vi "LEDExecute.vi"() -> ()   [LabVIEW 2023]
uses:
  <vilib>/Rock Robotics/WPI/DriverStation/WPI_DriverStationAllianceInfo.ctl
  Human/HumanGlobal.vi
  <vilib>/Rock Robotics/WPI/ThirdParty/PhotonVisionLib/PhotonVisionLib.lvlib
panel:
  out "Numeric":i32
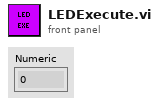
[diagram p1: front panel]
types:
  T1 = typedef "WPI_DriverStationAllianceInfo.ctl" = enum16{"Red", "Blue", "Invalid"}
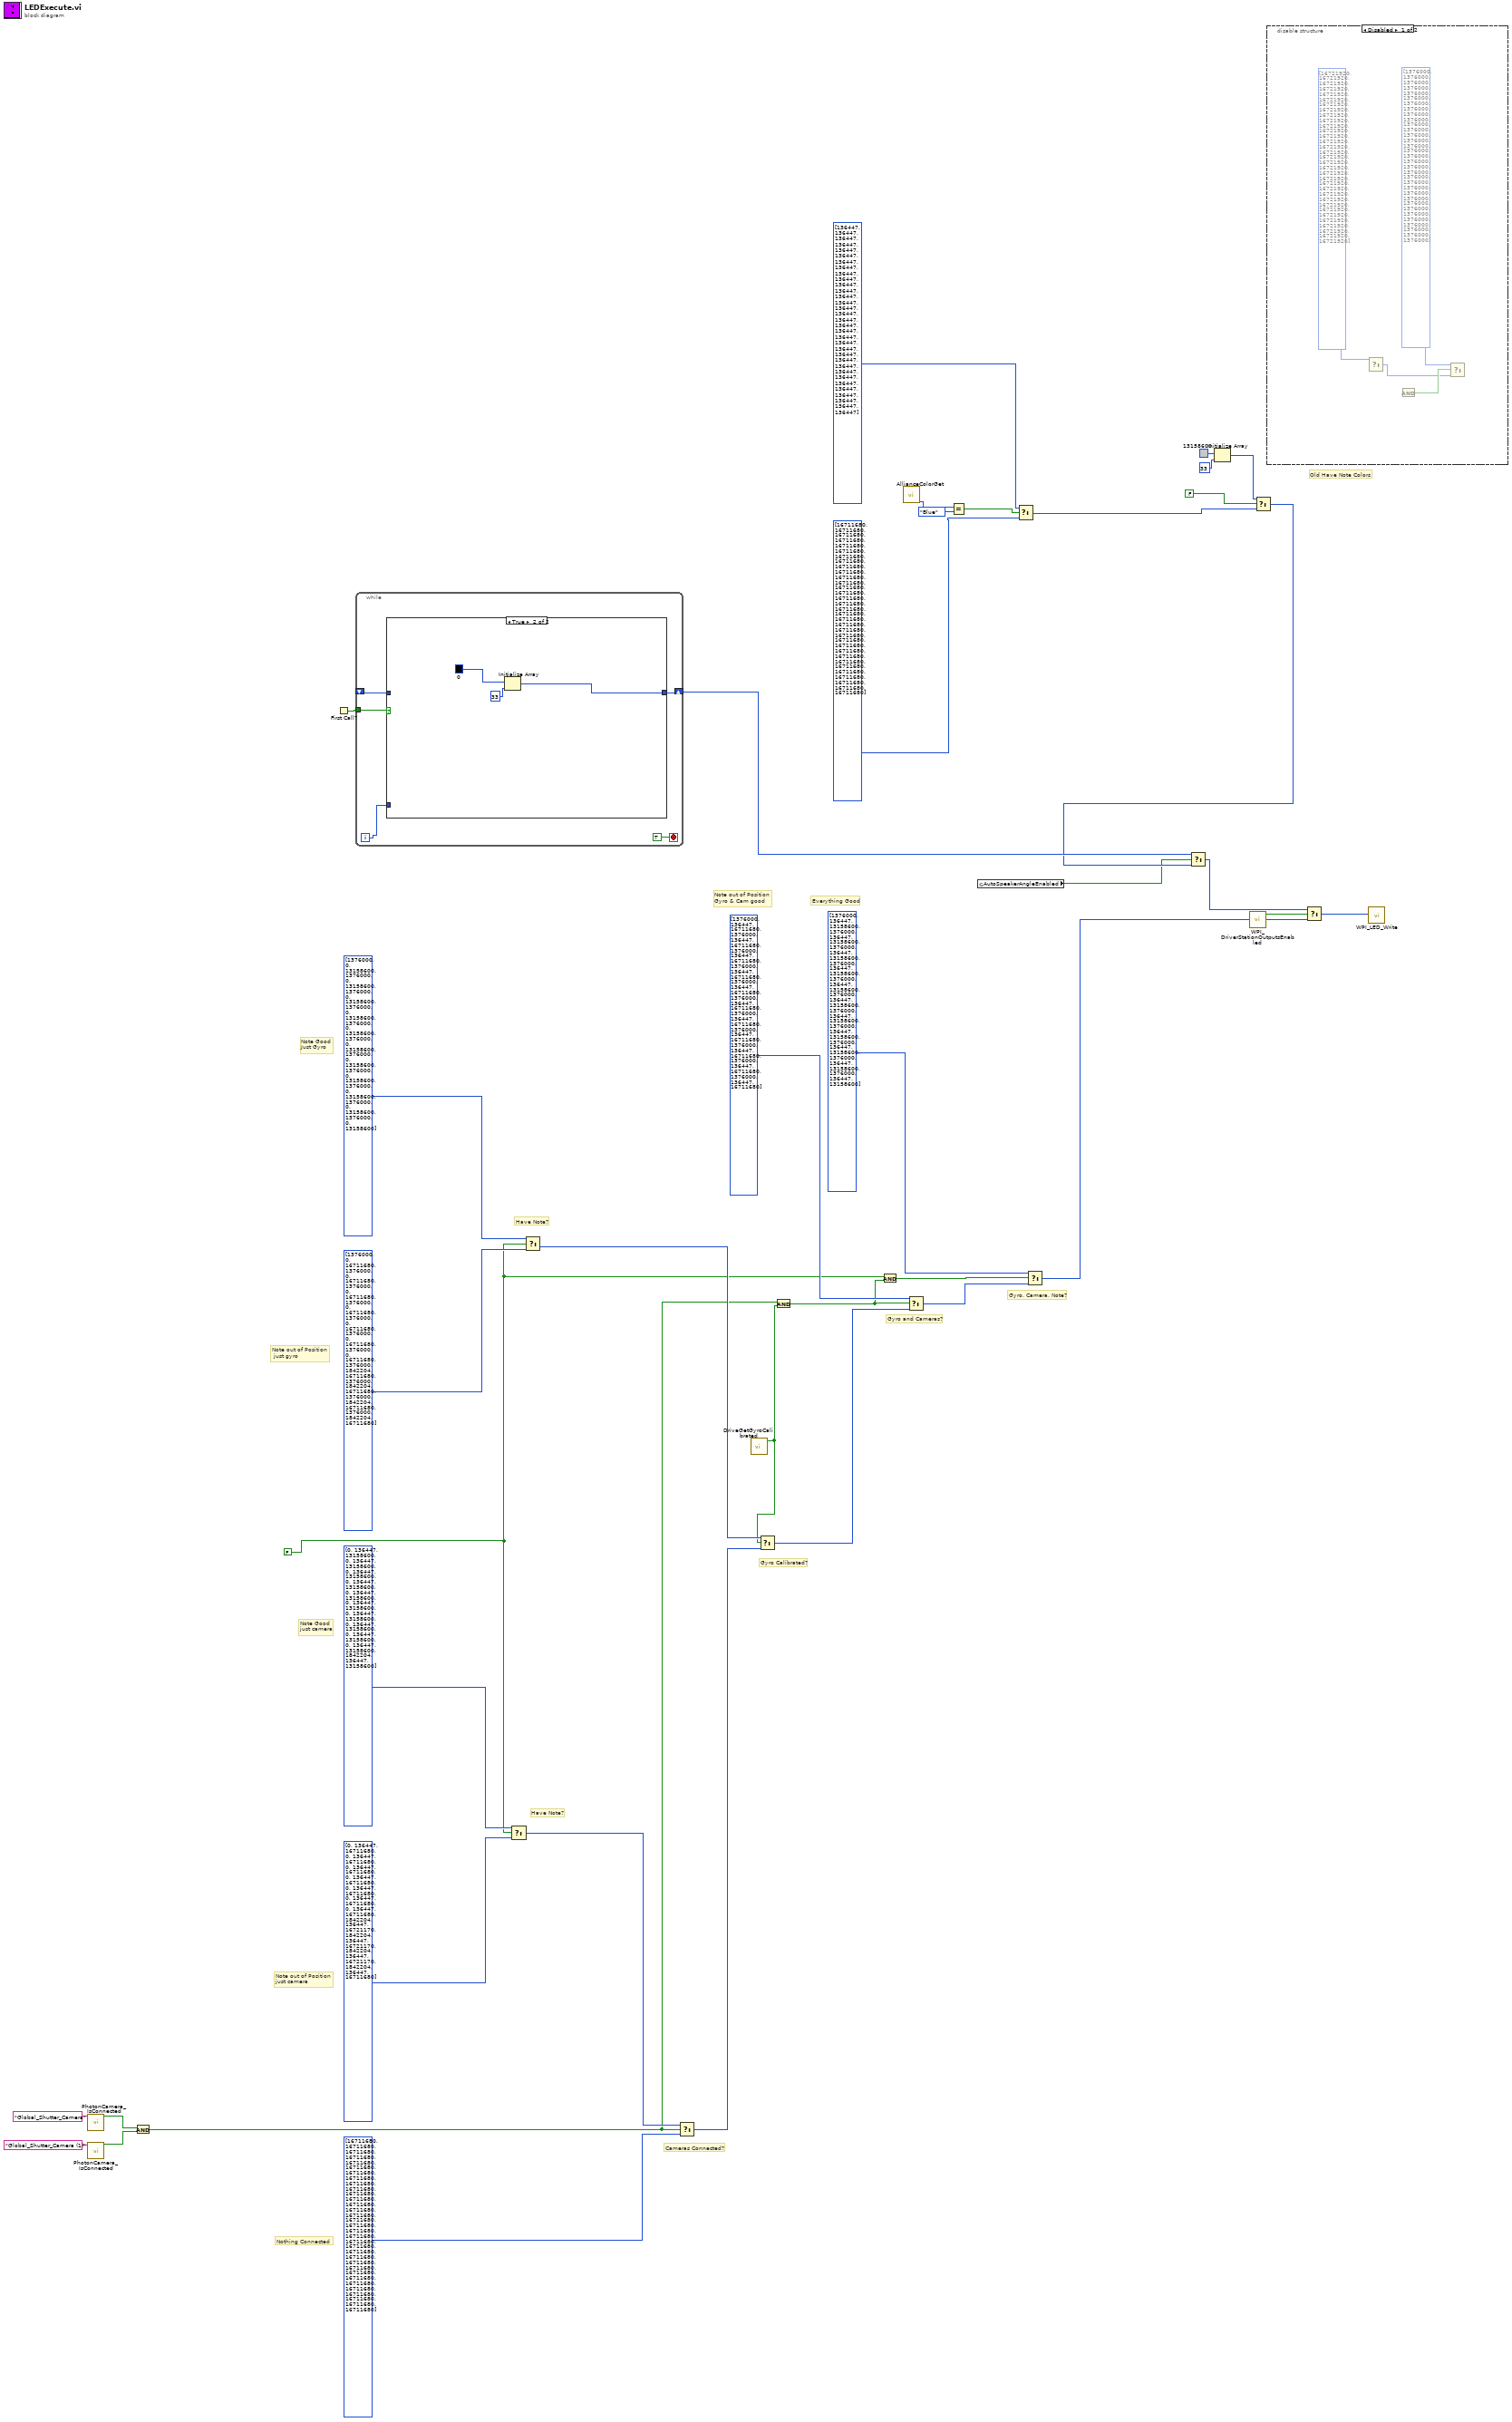
[diagram p0: block diagram]
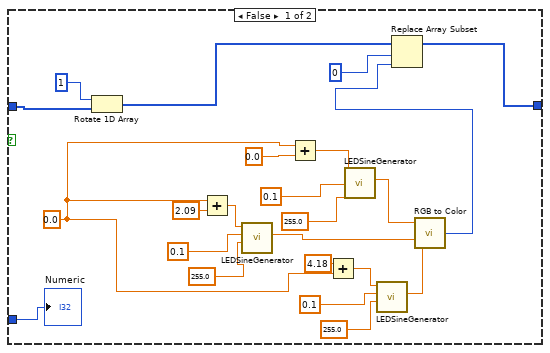
[diagram p2: hidden frame]
diagram:
  w1 = FALSE ("s")
  # "Old Have Note Colors"
  # "Gyro, Camera, Note?"
  # "Gyro and Cameras?"
  # "Gyro Calibrated?"
  # "Cameras Connected?"
  # "Have Note?"
  # "Have Note?"
  # "Note Good\njust camera"
  # "Note Good\nJust Gyro"
  # "Note out of Position\n just gyro"
  # "Note out of Position\njust camera"
  # "Everything Good"
  # "Note out of Position\nGyro & Cam good"
  # "Nothing Connected"
  n1 = call <vilib>:"PhotonCamera_IsConnected.vi"("CameraName"="Global_Shutter_Camera") -> ("IsConnected"=w20:bool)  [unwired: 9 in, 1 out]
  n2 = call <vilib>:"PhotonCamera_IsConnected.vi"("CameraName"="Global_Shutter_Camera (1)") -> ("IsConnected"=w19:bool)  [unwired: 9 in, 1 out]
  n3 = And(x=w20, y=w19) -> (x .and. y?=w23:bool)
  n4 = First Call?() -> (First Call?: T/F=w11:bool)
  n5 = while {
    tunnel: w11 -> [w43]
    shift-right: [w42] -> w9
    shift-left: _ -> [w41]
    i -> [w40]
    stop <- TRUE stop-if-true
    n6 = case shown="True" w43 {
      tunnel: [w58 w68] -> w42
      tunnel: w41 -> [w67 _]
      tunnel: w40 -> [w57 _]
      frame False {
        w61 = 0.0
        n7 = Rotate 1D Array(1:w67, 2:1 ("n")) -> (0:w65:u32[])
        n8 = Add(x=w61, y=2.09 ("Speed")) -> (x+y=w52:dbl)
        n9 = call "LEDSineGenerator.vi"("Amplitude"=255.0, "Speed"=0.1 ("Delay"), "Delay"=w52) -> ("Output"=w49:dbl)  [unwired: 8 in]
        n10 = Add(x=w61, y=0.0 ("Speed")) -> (x+y=w56:dbl)
        n11 = Add(x=4.18 ("Speed"), y=w61) -> (x+y=w48:dbl)
        n12 = call "LEDSineGenerator.vi"("Amplitude"=255.0, "Speed"=0.1 ("Delay"), "Delay"=w56) -> ("Output"=w53:dbl)  [unwired: 8 in]
        n13 = call "LEDSineGenerator.vi"("Amplitude"=255.0, "Speed"=0.1 ("Delay"), "Delay"=w48) -> ("Output"=w45:dbl)  [unwired: 8 in]
        n14 = call <vilib>:"RGB to Color.vi"("B"=w45, "G"=w49, "R"=w53) -> ("Color"=w60:u32)
        n15 = Replace Array Subset(array=w65, new element=w60, index=0) -> (w58:u32[])
        "Numeric" <- w57
      }
      frame True {
        n16 = Initialize Array(u32 0 ("Color Box 3"), 33 ("dimension size")) -> (w68:u32[])
      }
    }
  }
  n17 = Select(t=u32[] [0, 136447, 13158600, 0, 136447, 13158600, 0, 136447, 13158600, 0, 136447, 13158600, 0, 136447, 13158600, 0, 136447, 13158600, 0, 136447, 13158600, 0, 136447, 13158600, 0, 136447, 13158600, 0, 136447, 13158600, 1842204, 136447, 13158600] ("Color Array"), s=w1, f=u32[] [0, 136447, 16711680, 0, 136447, 16711680, 0, 136447, 16711680, 0, 136447, 16711680, 0, 136447, 16711680, 0, 136447, 16711680, 0, 136447, 16711680, 1842204, 136447, 16721170, 1842204, 136447, 16721170, 1842204, 136447, 16721170, 1842204, 136447, 16711680] ("Color Array")) -> (s? t:f=w32:u32[])
  n18 = Select(t=u32[] [1376000, 0, 13158600, 1376000, 0, 13158600, 1376000, 0, 13158600, 1376000, 0, 13158600, 1376000, 0, 13158600, 1376000, 0, 13158600, 1376000, 0, 13158600, 1376000, 0, 13158600, 1376000, 0, 13158600, 1376000, 0, 13158600, 1376000, 0, 13158600] ("Color Array"), s=w1, f=u32[] [1376000, 0, 16711680, 1376000, 0, 16711680, 1376000, 0, 16711680, 1376000, 0, 16711680, 1376000, 0, 16711680, 1376000, 0, 16711680, 1376000, 0, 16711680, 1376000, 1842204, 16711680, 1376000, 1842204, 16711680, 1376000, 1842204, 16711680, 1376000, 1842204, 16711680] ("Color Array")) -> (s? t:f=w34:u32[])
  n19 = Select(t=w32, s=w23, f=u32[] [16711680, 16711680, 16711680, 16711680, 16711680, 16711680, 16711680, 16711680, 16711680, 16711680, 16711680, 16711680, 16711680, 16711680, 16711680, 16711680, 16711680, 16711680, 16711680, 16711680, 16711680, 16711680, 16711680, 16711680, 16711680, 16711680, 16711680, 16711680, 16711680, 16711680, 16711680, 16711680, 16711680] ("Color Array")) -> (s? t:f=w39:u32[])
  n20 = call "DriveGetGyroCalibrated.vi"() -> ("GryoCalibrated"=w18:bool)  [unwired: 11 in]
  n21 = Select(t=w34, s=w18, f=w39) -> (s? t:f=w37:u32[])
  n22 = And(x=w23, y=w18) -> (x .and. y?=w25:bool)
  n23 = And(x=w1, y=w25) -> (x .and. y?=w24:bool)
  n24 = call "AllianceColorGet.vi"() -> ("AllianceColor"=w17:T1)  [unwired: 11 in]
  n25 = Select(t=u32[] [1376000, 136447, 16711680, 1376000, 136447, 16711680, 1376000, 136447, 16711680, 1376000, 136447, 16711680, 1376000, 136447, 16711680, 1376000, 136447, 16711680, 1376000, 136447, 16711680, 1376000, 136447, 16711680, 1376000, 136447, 16711680, 1376000, 136447, 16711680, 1376000, 136447, 16711680] ("Color Array"), s=w25, f=w37) -> (s? t:f=w29:u32[])
  n26 = Equal?(x=w17, y=WPI_DriverStationAllianceInfo."Blue") -> (x = y?=w13:bool)
  n27 = global read "HumanGlobal.vi" "AutoSpeakerAngleEnabled"() -> (w3:bool)
  n28 = Select(t=u32[] [136447, 136447, 136447, 136447, 136447, 136447, 136447, 136447, 136447, 136447, 136447, 136447, 136447, 136447, 136447, 136447, 136447, 136447, 136447, 136447, 136447, 136447, 136447, 136447, 136447, 136447, 136447, 136447, 136447, 136447, 136447, 136447, 136447] ("Color Array"), s=w13, f=u32[] [16711680, 16711680, 16711680, 16711680, 16711680, 16711680, 16711680, 16711680, 16711680, 16711680, 16711680, 16711680, 16711680, 16711680, 16711680, 16711680, 16711680, 16711680, 16711680, 16711680, 16711680, 16711680, 16711680, 16711680, 16711680, 16711680, 16711680, 16711680, 16711680, 16711680, 16711680, 16711680, 16711680] ("Color Array")) -> (s? t:f=w10:u32[])
  n29 = Select(t=u32[] [1376000, 136447, 13158600, 1376000, 136447, 13158600, 1376000, 136447, 13158600, 1376000, 136447, 13158600, 1376000, 136447, 13158600, 1376000, 136447, 13158600, 1376000, 136447, 13158600, 1376000, 136447, 13158600, 1376000, 136447, 13158600, 1376000, 136447, 13158600, 1376000, 136447, 13158600] ("Color Array"), s=w24, f=w29) -> (s? t:f=w28:u32[])
  n30 = Initialize Array(u32 13158600 ("Color Box 3"), 33 ("dimension size")) -> (w4:u32[])
  n31 = call <vilib>:"WPI_DriverStationOutputsEnabled.vi"() -> ("OutputsEnabled?"=w36:bool)  [unwired: 10 in, 1 out]
  n32 = Select(t=w4, s=FALSE, f=w10) -> (s? t:f=w8:u32[])
  n33 = Select(t=w9, s=w3, f=w8) -> (s? t:f=w7:u32[])
  n34 = disable-structure shown="Disabled" {
    frame Disabled {
      n35 = Select(t=u32[] [16721920, 16721920, 16721920, 16721920, 16721920, 16721920, 16721920, 16721920, 16721920, 16721920, 16721920, 16721920, 16721920, 16721920, 16721920, 16721920, 16721920, 16721920, 16721920, 16721920, 16721920, 16721920, 16721920, 16721920, 16721920, 16721920, 16721920, 16721920, 16721920, 16721920, 16721920, 16721920, 16721920] ("Color Array")) -> (s? t:f=w71:u32[])  [unwired: 2 in]
      n36 = And() -> (x .and. y?=w72:bool)  [unwired: 2 in]
      n37 = Select(t=u32[] [1376000, 1376000, 1376000, 1376000, 1376000, 1376000, 1376000, 1376000, 1376000, 1376000, 1376000, 1376000, 1376000, 1376000, 1376000, 1376000, 1376000, 1376000, 1376000, 1376000, 1376000, 1376000, 1376000, 1376000, 1376000, 1376000, 1376000, 1376000, 1376000, 1376000, 1376000, 1376000, 1376000] ("Color Array"), s=w72, f=w71) -> ()  [unwired: 1 out]
    }
    frame Enabled {
    }
  }
  n38 = Select(t=w7, s=w36, f=w28) -> (s? t:f=w12:u32[])
  n39 = call <vilib>:"WPI_LED_Write.vi"("Color Array"=w12) -> ()  [unwired: 10 in, 1 out]
